vi "Open Connection_TangentForcesMeasured.vi"(8 "error in (no error)":errorcluster, 9 "TangentForcesMeasured":T1, 10 "topicName":string) -> (0 "error out":errorcluster, 3 "topicRef":cluster{"topicName":string, "type":refnum<vi>})   [LabVIEW 2015]
uses:
  SALTypedefs/m2ms/TangentForcesMeasured.ctl
  SALTypedefs/m2ms/m2ms.lvlib
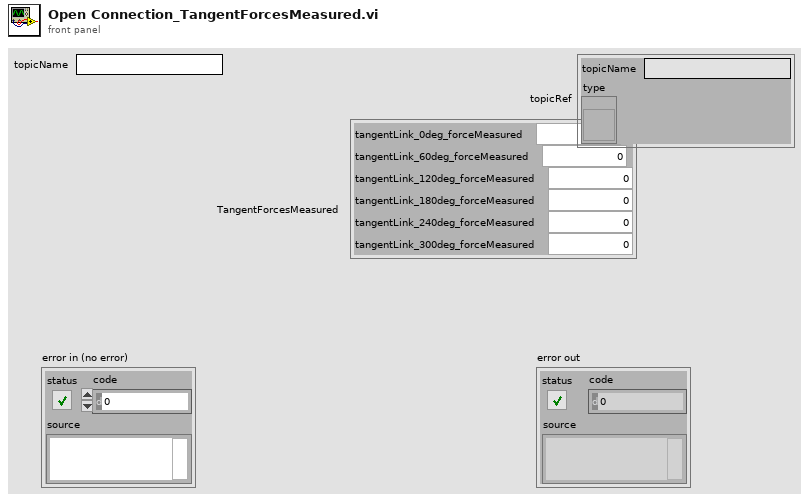
[diagram p1: front panel]
types:
  T1 = typedef "m2ms.lvlib/TangentForcesMeasured.ctl" = cluster{"tangentLink_0deg_forceMeasured":dbl, "tangentLink_60deg_forceMeasured":dbl, "tangentLink_120deg_forceMeasured":dbl, "tangentLink_180deg_forceMeasured":dbl, "tangentLink_240deg_forceMeasured":dbl, "tangentLink_300deg_forceMeasured":dbl}
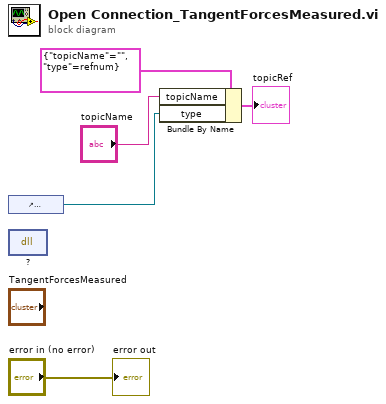
[diagram p0: block diagram]
diagram:
  n1 = control-ref of="TangentForcesMeasured"() -> (w2:refnum<vi>)
  n2 = dll-call lib="?" fn="?"() -> ()  [unwired: 4 in, 2 out]
  n3 = Bundle By Name(cluster=cluster{"topicName":string, "type":refnum<vi>} {"topicName"="", "type"=refnum} ("topicRef"), "topicName"="topicName", "type"=w2) -> (→"topicRef":cluster{"topicName":string, "type":refnum<vi>})
  "error out" <- "error in (no error)"
